vi "Servo MSMT TDSCDMA Set DC Params.vi"(8 "error in (no error)":errorcluster, 10 "Step In":refnum<k7>, 11 "Servo MSMT in":refnum<class "Servo MSMT.lvclass">) -> (0 "error out":errorcluster, 2 "Step Out":refnum<k7>, 3 "Servo MSMT out":refnum<class "Servo MSMT.lvclass">)   [LabVIEW 2018, in "Servo MSMT.lvlib" / "Servo MSMT.lvclass"]
uses:
  Servo MSMT.lvclass
  C:/Sequence Automation/Plugins/Measurement Interface.lvlibp/Measurement Interface.lvclass
  Servo MSMT.lvclass/Servo MSMT.ctl
  Protected Methods/Read DC Pins.vi
  Plugins/Measurement Interface.lvlibp/Private Methods/Engine Reference/Read Engine Reference.vi
  Plugins/TestStand API Tools (TSAT).lvlibp/Step Actions/TSAT Step Actions.lvlib
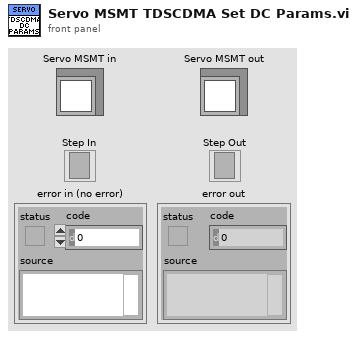
[diagram p1: front panel]
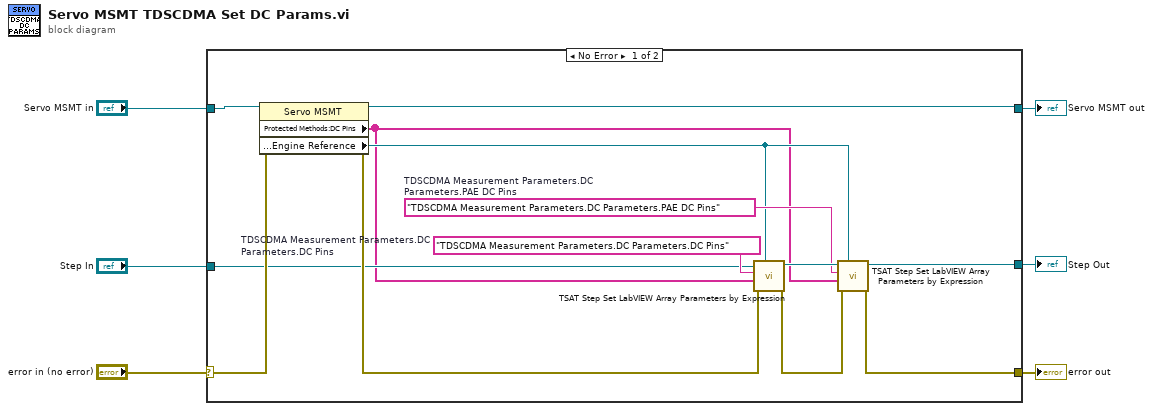
[diagram p0: block diagram]
diagram:
  n1 = case shown="No Error" "error in (no error)" {
    selector: "error in (no error)" -> [w19 w22]
    tunnel: [w13 w22] -> w5
    tunnel: [w17 w21] -> w3
    tunnel: "Servo MSMT in" -> [w18 w21]
    tunnel: "Step In" -> [w11 w20]
    tunnel: [w10 w20] -> w1
    frame No Error {
      w9 = "TDSCDMA Measurement Parameters.DC Parameters.PAE DC Pins"  # TDSCDMA Measurement Parameters.DC Parameters.PAE DC Pins
      w15 = "TDSCDMA Measurement Parameters.DC Parameters.DC Pins"  # TDSCDMA Measurement Parameters.DC Parameters.DC Pins
      n2 = property class="Servo MSMT"(reference=w18, error in=w19) -> (reference out=w17:refnum<class "Servo MSMT.lvclass">, error out=w16:errorcluster, "Protected Methods:DC Pins"=w7:string[], "Protected Methods:Engine Reference"=w8:refnum<k7>)
      n3 = call "TSAT Step Set LabVIEW Array Parameters by Expression.vi"("Engine In"=w8, "Error In"=w16, "Value Expressions"=w7, "Parameter to Set"=w15, "Step In"=w11) -> ("Error Out"=w14:errorcluster, "Step Out"=w12:refnum<k7>)  [unwired: 5 in]
      n4 = call "TSAT Step Set LabVIEW Array Parameters by Expression.vi"("Engine In"=w8, "Error In"=w14, "Value Expressions"=w7, "Parameter to Set"=w9, "Step In"=w12) -> ("Error Out"=w13:errorcluster, "Step Out"=w10:refnum<k7>)  [unwired: 5 in]
    }
    frame Error {
    }
  }
  "error out" <- w5
  "Servo MSMT out" <- w3
  "Step Out" <- w1
